vi "Launch Nested with API.vi"(7 "API Type":refnum<class "API.lvclass">, 8 "error in (no error)":errorcluster, 10 "Nested Task":refnum<class "Task.lvclass">, 11 "Task in":refnum<class "Task.lvclass">) -> (0 "error out":errorcluster, 2 "API":refnum<class "API.lvclass">, 3 "Task out":refnum<class "Task.lvclass">)   [LabVIEW 2020, in "Volatus.lvlib" / "Task.lvclass"]
uses:
  Task.lvclass
  API/API.lvclass
  API Provider/API Provider.lvclass
  lv-promises/Promises/Promise/Promise.lvclass/Promise.ctl
  lv-promises/Promises/Future/Future.lvclass/Future.ctl
  API Provider Messages/Request API Msg/Request API Msg.lvclass/Request API Msg.ctl
  <vilib>/ActorFramework/Message Enqueuer/Message Enqueuer.lvclass/Message Enqueuer.ctl
  API Provider Messages/Request API Msg/Send Request API.vi
  lv-promises/Promises/Promise/Future.vi
  <vilib>/ActorFramework/Message Enqueuer/Enqueue.vi
  lv-promises/Promises/Future/Create.vi
  ApiValue/ApiValue.lvclass
  C:/dev/lv20CE/relink/lv-promises/Promises/Value/Value.lvclass
  API Provider Messages/Request API Msg/Request API Msg.lvclass
  C:/Program Files (x86)/National Instruments/LabVIEW 2020/vi.lib/ActorFramework/Message/Message.lvclass
  lv-promises/Promises/Promise/Create.vi
  <vilib>/ActorFramework/Message Priority Queue/Priority Enqueue.vi
  lv-promises/Promises/Future/Wait.vi
  ApiValue/Read.vi
  <vilib>/ActorFramework/Message Enqueuer/Message Enqueuer.lvclass
  lv-promises/Promises/Future/Future.lvclass
  Task.lvclass/Task.ctl
  Volatus.lvlib
  C:/Program Files (x86)/National Instruments/LabVIEW 2020/vi.lib/ActorFramework/Actor/Actor.lvclass
  C:/dev/lv20CE/relink/lv-volatus/Volatus/Task/Task.lvclass
  C:/dev/lv20CE/relink/lv-volatus/Volatus/APIRegistrationHandler/APIRegistrationHandler.lvclass
  C:/dev/lv20CE/relink/lv-volatus/Volatus/TaskStateHandler/TaskStateHandler.lvclass
  C:/dev/lv20CE/relink/lv-volatus/Volatus/VectoMessageHandler/VectoMessageHandler.lvclass
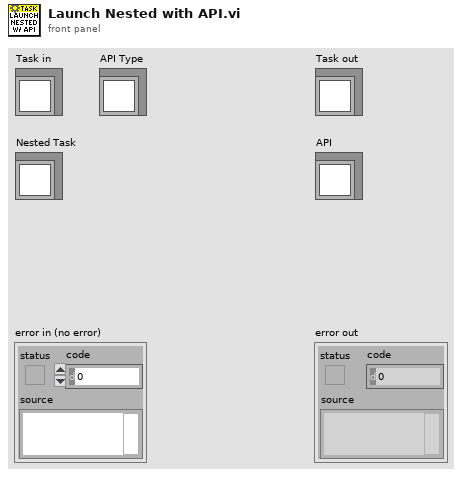
[diagram p1: front panel]
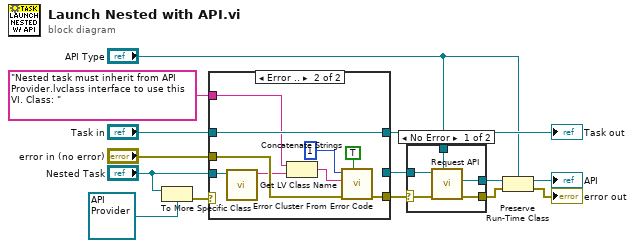
[diagram p0: block diagram]
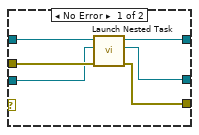
[diagram p2: hidden frame]
diagram:
  n1 = To More Specific Class(target class=refnum<class "API Provider.lvclass"> refnum ("Volatus:API Provider.lvclass"), reference="Nested Task") -> (error out=w6:errorcluster)  [unwired: 1 in, 1 out]
  n2 = case shown="Error .." w6 {
    tunnel: "error in (no error)" -> [w20 w29]
    tunnel: "Task in" -> [w19 w28]
    tunnel: [w18 w28] -> w12
    tunnel: [w17 w27] -> w10
    tunnel: [w16 _] -> w9
    tunnel: "Nested Task" -> [w15 w24]
    tunnel: "Nested task must inherit from API Provider.lvclass interface to use this VI. Class: " -> [_ w22]
    frame No Error {
      n3 = call "Launch Nested Task.vi"("error in (no error)"=w20, "Nested Task"=w15, "Task in"=w19) -> ("error out"=w17:errorcluster, "Nested EnQr"=w16:refnum<class "Message Enqueuer.lvclass">, "Task out"=w18:refnum<class "Task.lvclass">)  [unwired: 6 in]
    }
    frame Error {
      n4 = call <vilib>:"Get LV Class Name.vi"("object"=w24) -> ("class name"=w23:string)  [unwired: 9 in, 1 out]
      n5 = Concatenate Strings(w22, w23) -> (w21:string)
      n6 = call <vilib>:"Error Cluster From Error Code.vi"("show call chain? (False)"=TRUE, "error in (no error)"=w29, "error message (\"\")"=w21, "error code (0)"=1) -> ("error out"=w27:errorcluster)  [unwired: 5 in]
    }
  }
  "Task out" <- w12
  n7 = case shown="No Error" w10 {
    selector: w10 -> [w32 w35]
    tunnel: "API Type" -> [w34 _]
    tunnel: [w33 _] -> w11
    tunnel: w9 -> [w31 _]
    tunnel: [w30 w35] -> w3
    frame No Error {
      n8 = call "Request API.vi"("API Type"=w34, "error in (no error)"=w32, "EnQr"=w31) -> ("error out"=w30:errorcluster, "API"=w33:refnum<class "API.lvclass">)  [unwired: 7 in]
    }
    frame Error {
    }
  }
  n9 = Preserve Run-Time Class(object in=w11, error in=w3, 2:"API Type") -> (object out=→"API":refnum<class "API.lvclass">, error out=→"error out":errorcluster)
